vi "ResetRequest.vi"(8 "ErrorArray In":errorcluster[](array[cluster]), 10 "clFrontPanelControlRefs":T1) -> (0 "ErrorArray Out":errorcluster[](array[cluster]))   [LabVIEW 2014, in "TestFramework.lvlib"]
uses:
  TestFramework.lvlib
  TypeDefs/clFrontPanelControlRefs.ctl
  FGenPlugins/MyPluginBaseClass/TypeDef/PluginParams.ctl
  WfrmGenerator/WfrmPlugins/EventPluginBaseClass/TypeDefs/dblEvtSignalArray.ctl
  FGenPlugins/MyPluginBaseClass/TypeDef/CreateArbWfrmParams.ctl
  WfrmGenerator/WfrmPlugins/EventPluginBaseClass/TypeDefs/clEvtConfig.ctl
  WfrmGenerator/WfrmModule/PublicAPI/Arguments/Requests/dblEvtParams.ctl
  FGenPlugins/MyPluginBaseClass/TypeDef/ConfigArbWfrmParams.ctl
  FGenPlugins/MyPluginBaseClass/TypeDef/TriggerParams.ctl
  Bus/NISTBus.lvclass
  FGenPlugins/MyPluginBaseClass/NISTFGenPluginsBase.lvclass
  WfrmGenerator/WfrmPlugins/EventPluginBaseClass/BaseWfrmPlugin.lvclass
  WfrmGenerator/WfrmModule/WfrmModule.lvlib
panel:
  # "When you add a control \non the front panel, add a\nreference for it in this\ntype def.  This cluster\nwill hold all of the refer-\nences to the front panel\ncontrols in order to pass\nthese control references \nto subvis."
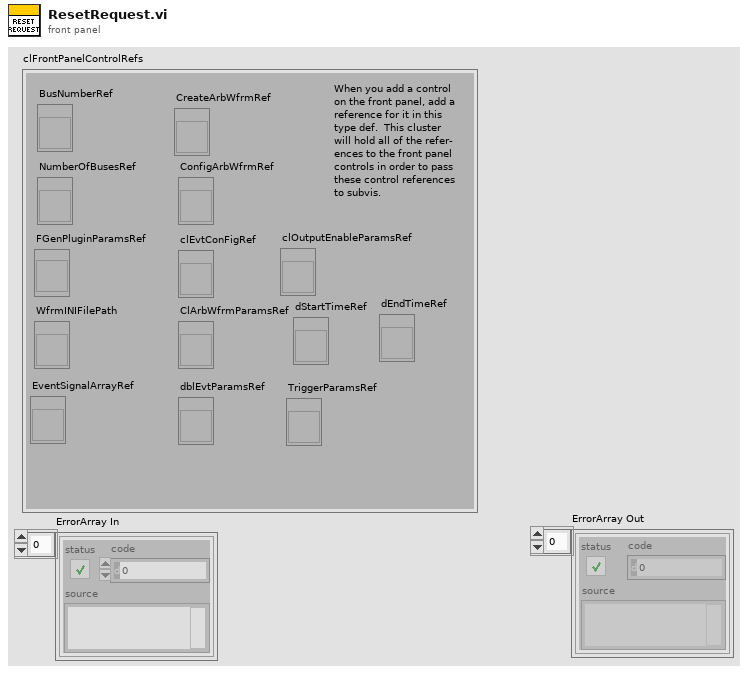
[diagram p1: front panel]
types:
  T1 = typedef "TestFramework.lvlib/clFrontPanelControlRefs.ctl" = cluster{"BusNumberRef":refnum<vi>, "NumberOfBusesRef":refnum<vi>, "FGenPluginParamsRef":refnum<vi>, "WfrmINIFilePath":refnum<vi>, "EventSignalArrayRef":refnum<vi>, "CreateArbWfrmRef":refnum<vi>, "clEvtConFigRef":refnum<vi>, "dblEvtParamsRef":refnum<vi>, "clOutputEnableParamsRef":refnum<vi>, "ConfigArbWfrmRef":refnum<vi>, "ClArbWfrmParamsRef":refnum<vi>, "dStartTimeRef":refnum<vi>, "dEndTimeRef":refnum<vi>, "TriggerParamsRef":refnum<vi>}
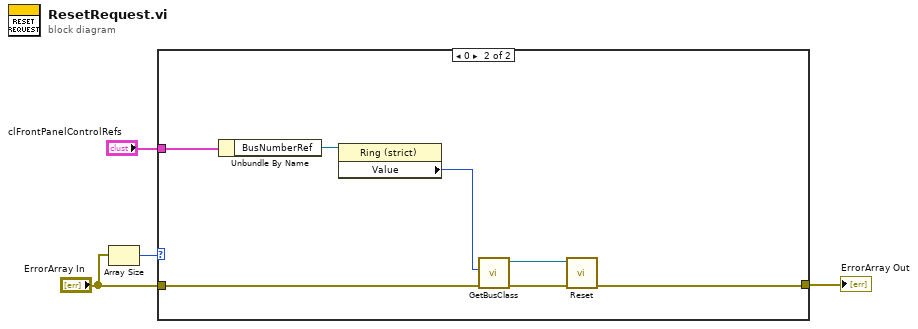
[diagram p0: block diagram]
diagram:
  n1 = Array Size(array="ErrorArray In") -> (size(s)=w4:i32)
  n2 = case shown="0" w4 {
    tunnel: "ErrorArray In" -> [w5 w11]
    tunnel: [w5 w8] -> w2
    tunnel: "clFrontPanelControlRefs" -> [_ w9]
    frame 1, Default {
    }
    frame 0 {
      n3 = Unbundle By Name(w9) -> ("BusNumberRef"=w12:refnum<vi>)
      n4 = property class="Ring (strict)"(reference=w12) -> ("Value"=w10:u8)  [unwired: 1 in, 2 out]
      n5 = call "GetBusClass.vi"("ErrorArray In"=w11, "BusNumber"=w10) -> ("ErrorArray Out"=w7:errorcluster[], "NISTBus Out"=w6:refnum<class "NISTBus.lvclass">)  [unwired: 8 in]
      n6 = call "Reset.vi"("ErrorArray In"=w7, "NISTBus In"=w6) -> ("ErrorArray Out"=w8:errorcluster[])  [unwired: 8 in, 1 out]
    }
  }
  "ErrorArray Out" <- w2
